vi "Create_Raw_data_file.vi"(4 "No of averages":i32=1, 5 "End time":dbl, 6 "Start time":dbl, 7 "Setup filename":string) -> (0 "Error String":string, 1 "Values":string[][](array[string]), 2 "Header Comments":string[](array[string]), 3 "Column headers":string[](array[string]))   [LabVIEW 2011]
uses:
  File/Setup_Filetype.ctl
  Controls/Post_Process.ctl
  Globals/Preference_global.vi
  Globals/Meas_global.vi
  Globals/Trav_pos_global.vi
  Globals/Constants_global.vi
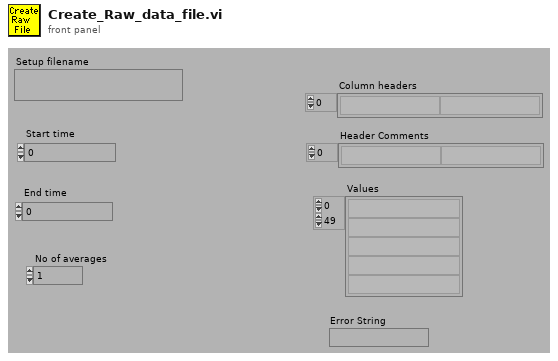
[diagram p1: front panel]
types:
  T1 = typedef "Post_Process.ctl" = enum16{"Take New Data", "Post Process Raw Data File"}
  T2 = typedef "Server_Comms.ctl" = enum16{"Server Link Healthy", "Do Not Link To Server"}
  T3 = typedef "Setup_Filetype.ctl" = enum16{"Measurement Setups", "Calibration Setups", "General", "Results File Plotter Setups", "Speed Calib Tweaks"}
  T4 = typedef "Traverse_cluster.ctl" = cluster{"Start X":dbl, "Start Y":dbl, "Start Z":dbl, "End X":dbl, "End Y":dbl, "End Z":dbl, "No. of pts.":i32, "Spacing":T5, "Filename":path, "Tunnel Speed":dbl, "Averaging time (min)":dbl, "Extra Commands":string, "Specific Arguments":string, "Emission Rate (l/min)":dbl, "Trace Gas Concentration (%)":dbl, "Density Ratio":string, "Comments":string, "Row No":i32, "Row Type Selector":T6, "Completion time":string, "Row Duration (mins)":dbl, "No. of Valid pts.":i32, "Meas Setup File":string}
  T5 = typedef "Spacing.ctl" = enum16{"Linear", "Log", "Gauss", "Specified", "N/A"}
  T6 = typedef "Multi_run_mode.ctl" = enum16{"Move Traverse Only", "Set Tunnel Speed Only", "Set Source Only", "Set Measurement Conditions", "Single Measurement", "Vertical Profile", "Lateral Profile", "Longitudinal Profile", "Explore Volume", "Multi-Axis Profile", "Auto Calibrate", "Meas Fast FID Bkgnd", "Check Beam Power", "Scanning Valve Measurement", "Run VI Named:", "Set ADAM Ch", "Wait (minutes)", "Send Message", "Synchronize With:", "Fall Back to this Row", "Turn Off Row Repeating", "Blank Row", "Traverse 3D Volume"}
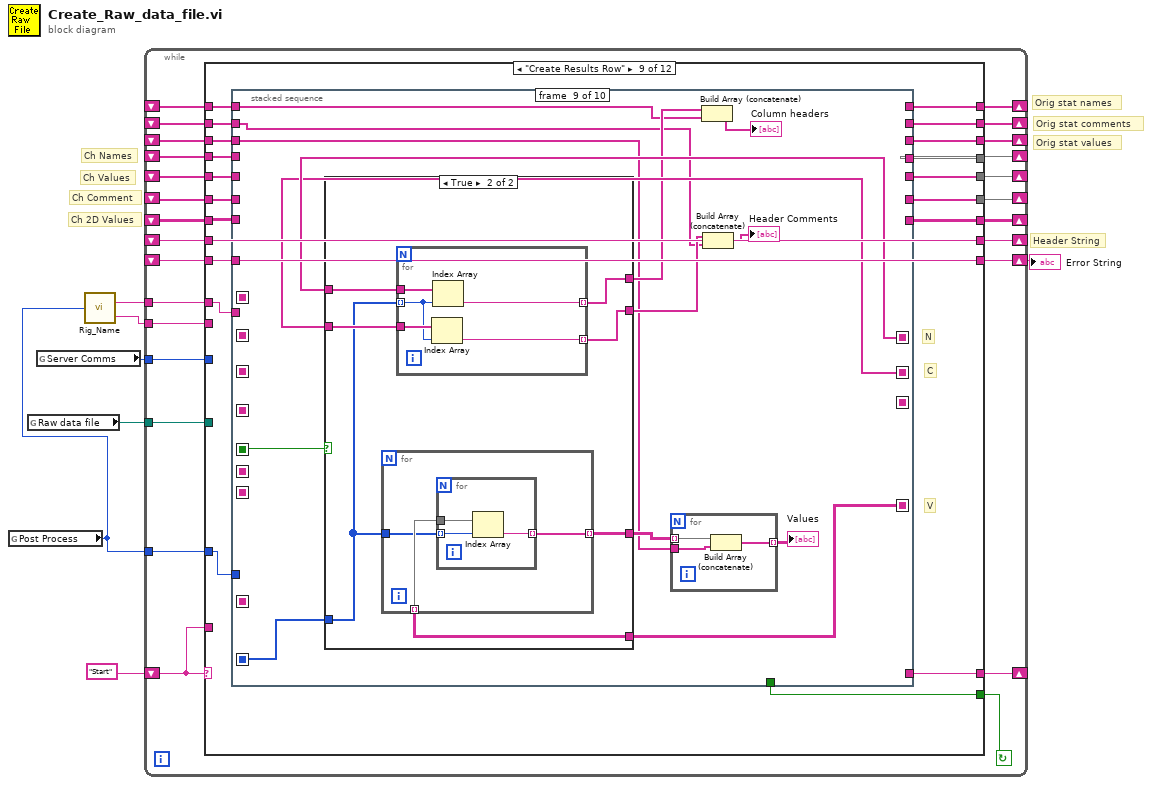
[diagram p0: block diagram]
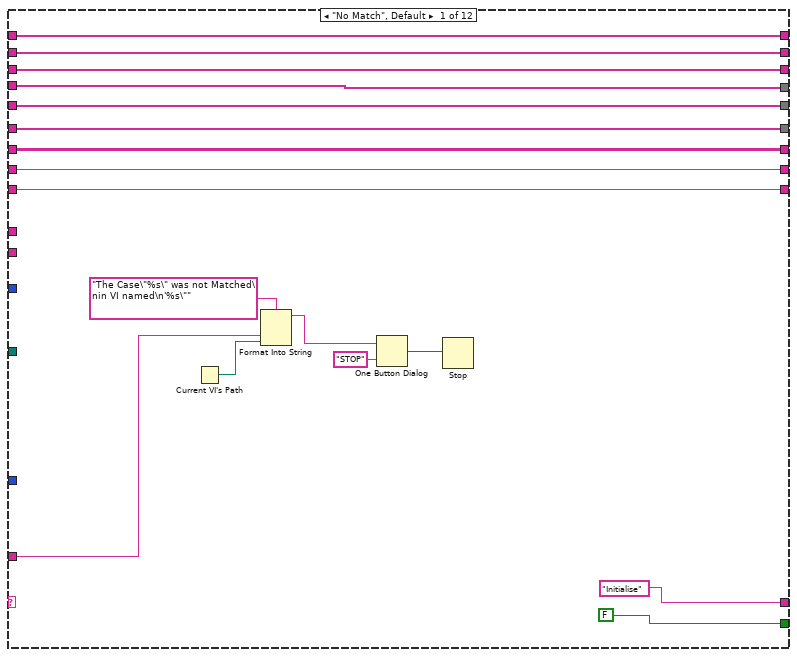
[diagram p2: hidden frame]
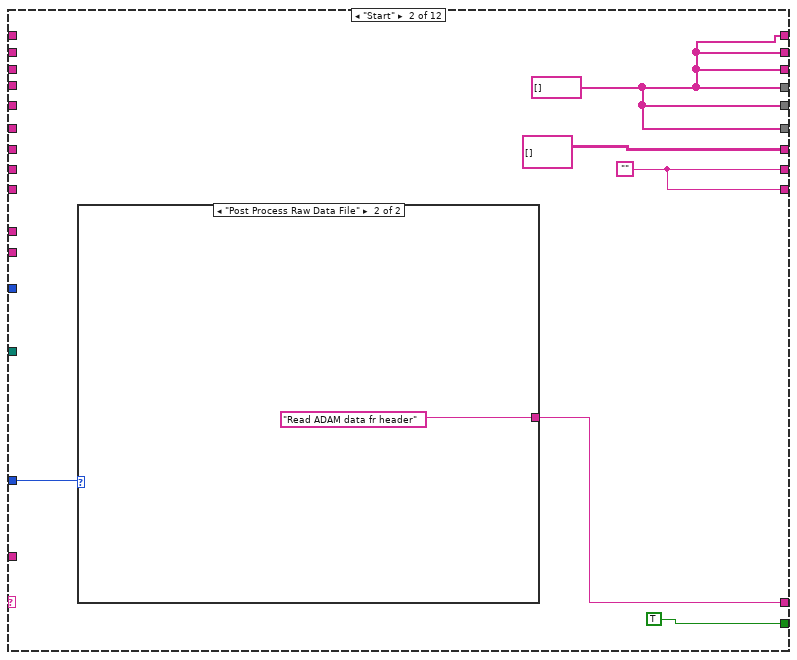
[diagram p3: hidden frame]
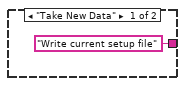
[diagram p4: hidden frame]
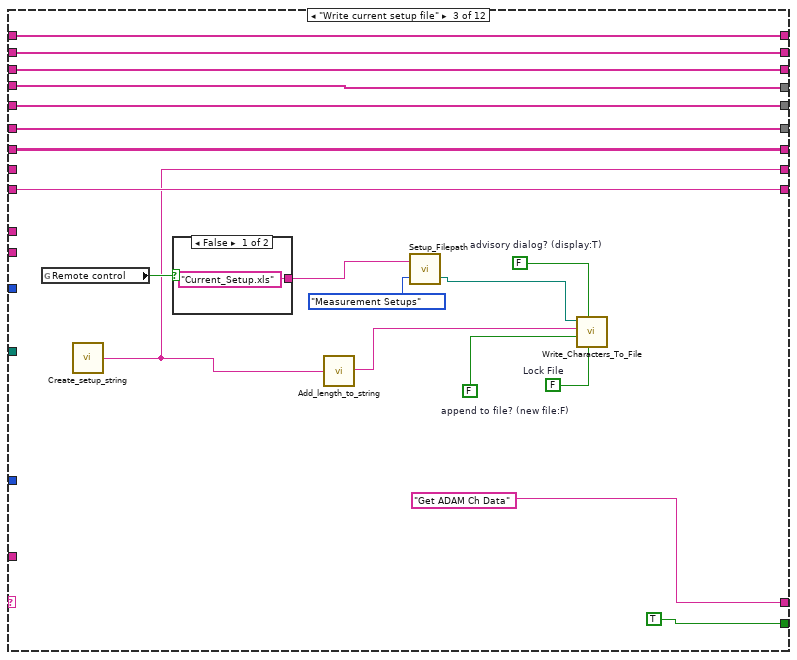
[diagram p5: hidden frame]
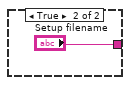
[diagram p6: hidden frame]
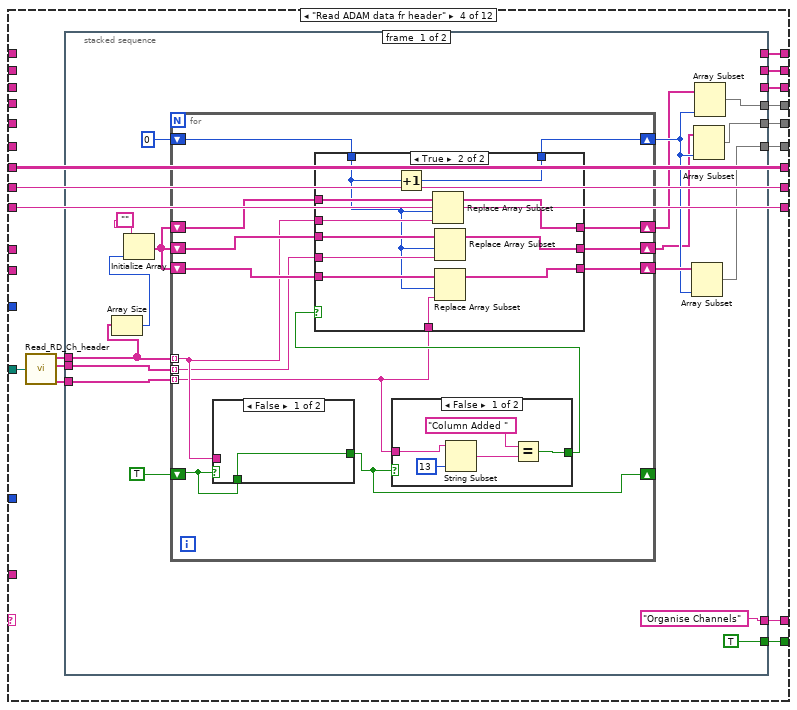
[diagram p7: hidden frame]
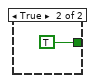
[diagram p9: hidden frame]
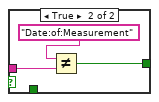
[diagram p10: hidden frame]
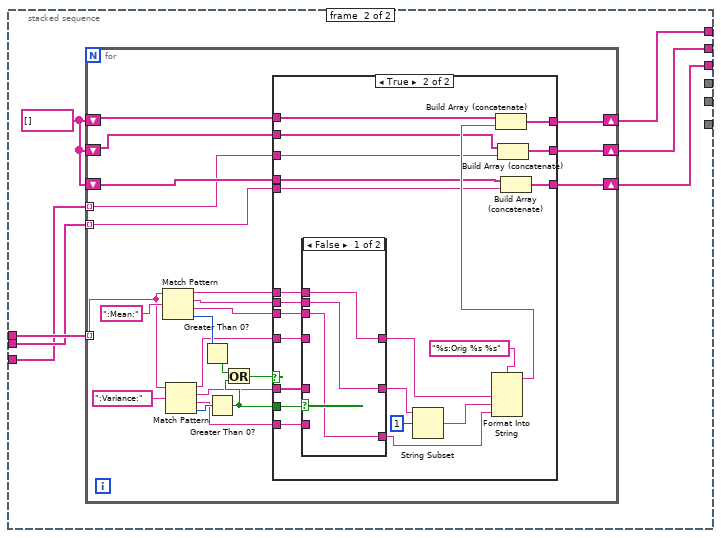
[diagram p11: hidden frame]
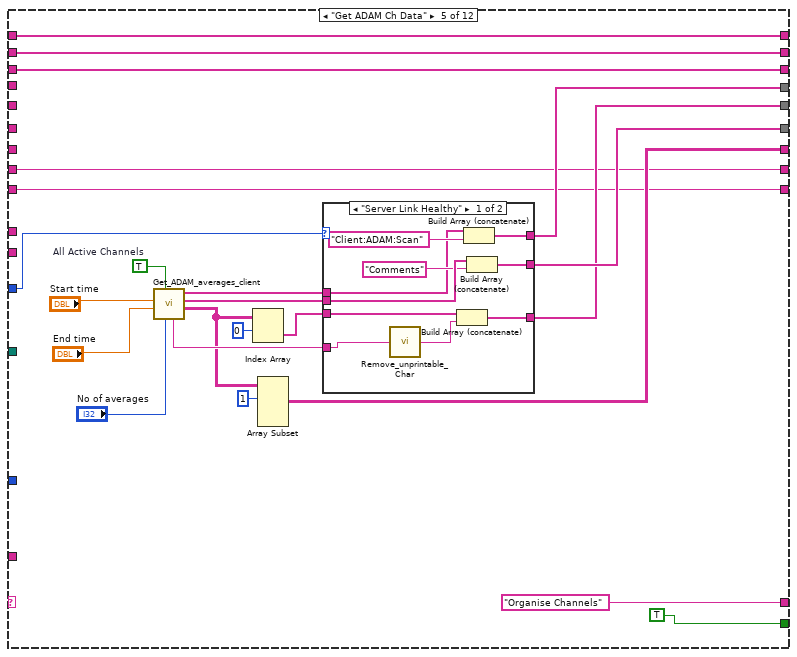
[diagram p14: hidden frame]
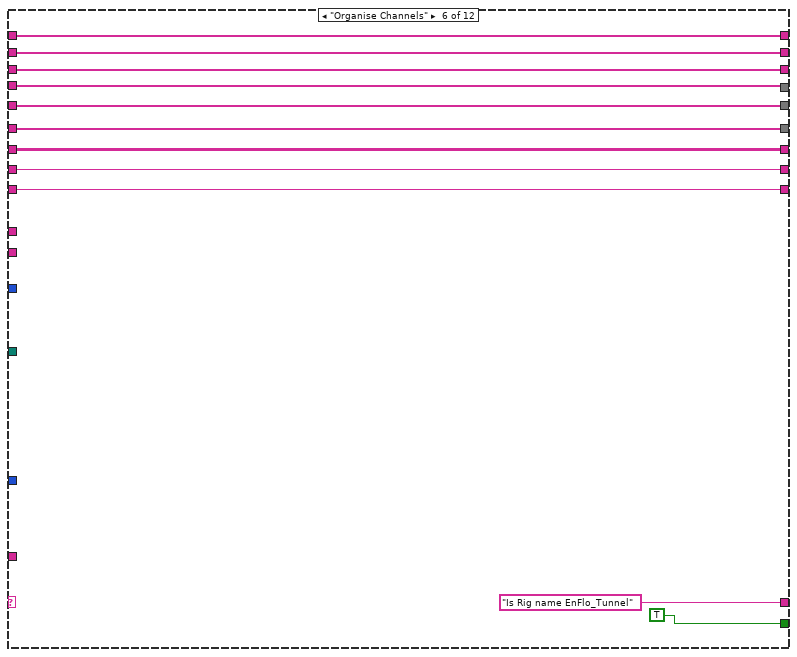
[diagram p16: hidden frame]
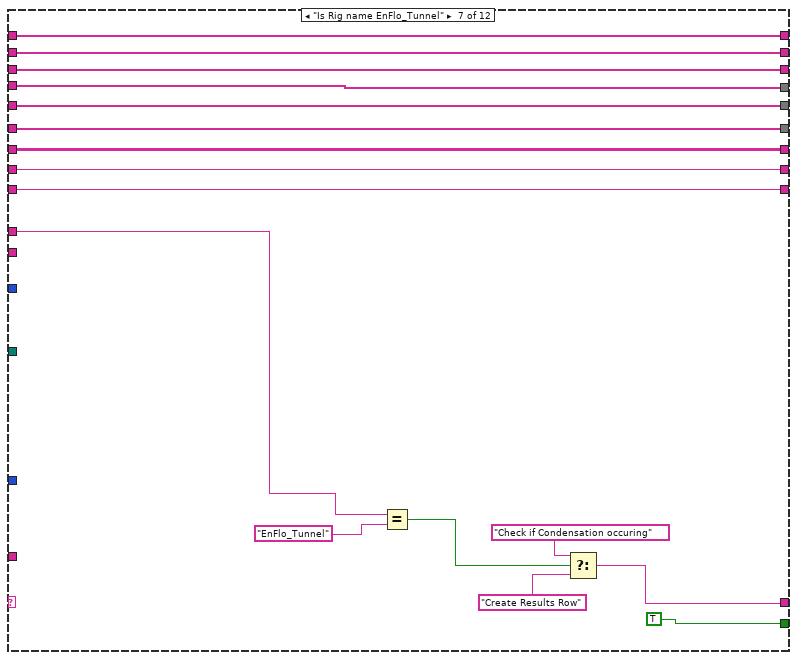
[diagram p17: hidden frame]
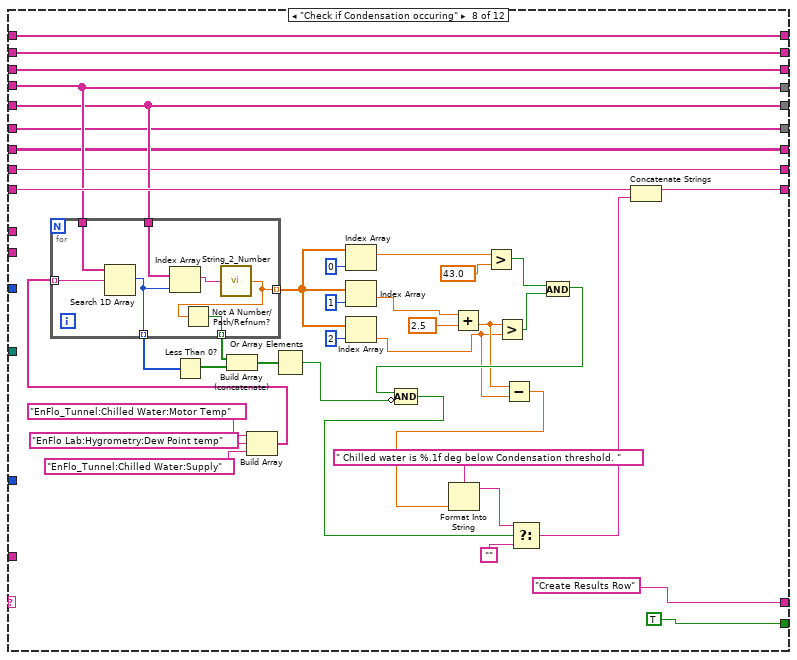
[diagram p18: hidden frame]
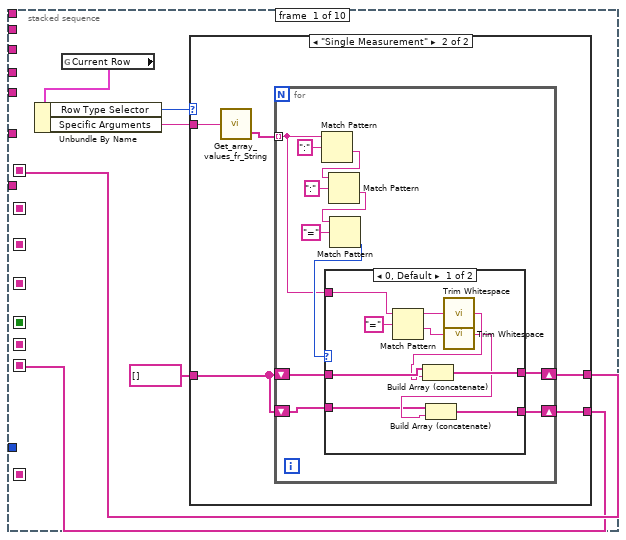
[diagram p19: hidden frame]
diagram:
  # "Orig stat values"
  # "Orig stat comments"
  # "Orig stat names"
  # "Header String"
  # "Ch 2D Values"
  # "Ch Comment"
  # "Ch Values"
  # "Ch Names"
  n1 = global read "Meas_global.vi" "Post Process"() -> (w3:T1)
  n2 = global read "Meas_global.vi" "Raw data file"() -> (w6:path)
  n3 = global read "Preference_global.vi" "Server Comms"() -> (w5:T2)
  n4 = call "Rig_Name.vi"("Post Process"=w3) -> ("Rig Setup before dash"=w2:string, "Hard Disk name"=w1:string)
  n5 = while {
    tunnel: w5 -> [w16]
    tunnel: w6 -> [w17]
    tunnel: w3 -> [w18]
    shift-left: _ -> [w20]
    shift-right: [w19] -> _
    shift-left: _ -> [w26]
    shift-right: [w25] -> w4
    shift-left: _ -> [w21]
    shift-right: [w27] -> _
    shift-left: _ -> [w22]
    shift-right: [w29] -> _
    shift-left: _ -> [w23]
    shift-right: [w28] -> _
    shift-left: _ -> [w24]
    shift-right: [w30] -> _
    shift-left: "Start" -> [w31]
    shift-right: [w32] -> _
    tunnel: w2 -> [w15]
    tunnel: w1 -> [w14]
    shift-right: [w10] -> _
    shift-left: _ -> [w11]
    shift-right: [w8] -> _
    shift-left: _ -> [w9]
    shift-right: [w12] -> _
    shift-left: _ -> [w13]
    stop <- w33 continue-if-true
    n6 = case shown="\"Create Results Row\"" w31 {
      tunnel: [FALSE TRUE TRUE w83 TRUE TRUE TRUE TRUE w328 TRUE TRUE FALSE] -> w33
      tunnel: ["Initialise" w52 "Get ADAM Ch Data" w94 "Organise Channels" "Is Rig name EnFlo_Tunnel" w265 "Create Results Row" w340 "Add Raw Data header info" "Add Raw Data fr Tempory file" "End"] -> w32
      tunnel: w31 -> [w45 _ _ _ _ _ _ _ _ _ _ _]
      tunnel: [w42 w51 w77 w85 w221 w255 w273 w283 w337 w625 w655 w672] -> w30
      tunnel: [w40 w51 w75 w86 w220 w253 w271 w281 w334 w636 w657 w674] -> w29
      tunnel: [w41 w51 w76 w84 w219 w254 w272 w282 w330 w637 w656 w673] -> w28
      tunnel: [w39 string[][] [] w74 w92 w217 w252 w270 w280 w332 w628 w658 w675] -> w27
      tunnel: w26 -> [w38 _ w72 w93 w216 w250 w267 w286 w338 w641 w659 w676]
      tunnel: [w38 w54 w72 w93 w216 w250 w267 w284 w338 w641 w659 w676] -> w25
      tunnel: w24 -> [w42 _ w77 _ _ w255 w273 w283 w336 w625 w655 w672]
      tunnel: w23 -> [w41 _ w76 _ _ w254 w272 w282 w331 w637 w656 w673]
      tunnel: w22 -> [w40 _ w75 _ _ w253 w271 w281 w335 w636 w657 w674]
      tunnel: w21 -> [w39 _ w74 w92 _ w252 w270 w280 w333 w628 w658 w675]
      tunnel: w20 -> [w37 _ _ w91 w215 w251 w268 w278 w339 w630 w652 w671]
      tunnel: [w37 w54 w66 w91 w215 w251 w268 w278 w339 w633 w651 ""] -> w19
      tunnel: w18 -> [_ w53 _ _ _ _ _ _ w329 _ _ _]
      tunnel: w17 -> [_ _ _ w90 _ _ _ _ _ _ _ w667]
      tunnel: w16 -> [_ _ _ _ w214 _ _ _ _ _ _ _]
      tunnel: w15 -> [_ _ _ _ _ _ w262 _ w327 _ _ _]
      tunnel: w14 -> [_ _ _ _ _ _ _ _ _ _ _ _]
      tunnel: w13 -> [w36 _ w64 _ w213 w249 w260 w277 w325 w622 w650 w664]
      tunnel: [w36 w51 w64 w82 w213 w249 w260 w277 w326 w622 w650 w664] -> w12
      tunnel: w11 -> [w35 _ w63 _ w212 w248 w259 w276 w324 w621 w649 w663]
      tunnel: [w35 w51 w63 w81 w212 w248 w259 w276 w323 w621 w649 w663] -> w10
      tunnel: w9 -> [w34 _ w62 _ w211 w247 w258 w275 w321 w620 w648 w662]
      tunnel: [w34 w51 w62 w80 w211 w247 w258 w275 w322 w620 w648 w662] -> w8
      frame "No Match", Default {
        n7 = Current VI's Path() -> (path=w44:path)
        n8 = Format Into String(format string="The Case\"%s\" was not Matched\nin VI named\n'%s\"" ("Format String"), w45, w44) -> (resulting string=w48:string)  [unwired: 2 in, 1 out]
        n9 = One Button Dialog(message=w48, button name ("OK")="STOP") -> (true=w46:bool)
        n10 = Stop(stop? (T)=w46) -> ()
      }
      frame "Start" {
        w54 = ""
        w51 = string[] []
        n11 = case shown="\"Post Process Raw Data File\"" w53 {
          tunnel: ["Write current setup file" "Read ADAM data fr header"] -> w52
          frame "Take New Data" {
          }
          frame "Post Process Raw Data File" {
          }
        }
      }
      frame "Write current setup file" {
        w67 = FALSE  # Lock File
        w70 = FALSE  # advisory dialog? (display:T)
        w71 = FALSE  # append to file? (new file:F)
        n12 = global read "Meas_global.vi" "Remote control"() -> (w69:bool)
        n13 = call "Create_setup_string.vi"() -> ("Setup String"=w66:string)  [unwired: 1 out]
        n14 = case shown="False" w69 {
          tunnel: ["Current_Setup.xls" ("Setup filename") "Setup filename"] -> w60
          frame False {
          }
          frame True {
          }
        }
        n15 = call "Add_length_to_string.vi"("String in"=w66) -> ("String out"=w68:string)
        n16 = call "Setup_Filepath.vi"("Setup File Type"=Setup_Filetype."Measurement Setups", "Filename in"=w60) -> ("Filename Out"=w59:path)  [unwired: 1 out]
        n17 = call "Write_Characters_To_File.vi"("file path (dialog if empty)"=w59, "advisory dialog? (display:T)"=w70, "character string"=w68, "append to file? (new file:F)"=w71, "Lock File"=w67) -> ()  [unwired: 4 out]
      }
      frame "Read ADAM data fr header" {
        n18 = call "Read_RD_Ch_header.vi"("Raw data file"=w90) -> ("Ch Name Out"=w88:string[], "Ch Values"=w87:string[], "Comments"=w89:string[])  [unwired: 1 out]
        n19 = stacked-sequence {
          tunnel: ["Organise Channels" _] -> w94
          tunnel: w89 -> [w109 w154]
          tunnel: w88 -> [w108 w157]
          tunnel: w87 -> [w103 w155]
          tunnel: [w100 _] -> w86
          tunnel: [w97 _] -> w85
          tunnel: [w96 _] -> w84
          tunnel: [TRUE _] -> w83
          tunnel: [_ w153] -> w82
          tunnel: [_ w152] -> w81
          tunnel: [_ w151] -> w80
          frame #0 {
            n20 = Array Size(array=w108) -> (size(s)=w106:i32)
            n21 = Initialize Array("", w106) -> (w105:string[])
            n22 = for {
              shift-right: [w112] -> w101
              shift-left: 0 -> [w122]
              shift-right: [w116] -> w102
              shift-left: w105 -> [w119]
              shift-right: [w117] -> w99
              shift-left: w105 -> [w120]
              shift-right: [w118] -> w98
              shift-left: w105 -> [w121]
              shift-right: [w124] -> _
              shift-left: TRUE -> [w125]
              tunnel: w108 -> [w115] mode=indexing
              tunnel: w109 -> [w113] mode=indexing
              tunnel: w103 -> [w114] mode=indexing
              n23 = case shown="False" w125 {
                tunnel: w115 -> [_ w150]
                tunnel: [w147 w148] -> w124
                tunnel: w125 -> [w147 _]
                frame False {
                }
                frame True {
                  n24 = Not Equal?(x="Date:of:Measurement", y=w150) -> (x != y?=w148:bool)
                }
              }
              n25 = case shown="False" w124 {
                tunnel: w113 -> [w142 _]
                tunnel: [w144 TRUE] -> w123
                frame False {
                  n26 = String Subset(string=w142, length (rest)=13 ("length (rest)")) -> (substring=w141:string)  [unwired: 1 out]
                  n27 = Equal?(x="Column Added ", y=w141) -> (x = y?=w144:bool)
                }
                frame True {
                }
              }
              n28 = case shown="True" w123 {
                tunnel: w122 -> [w126 w131]
                tunnel: w121 -> [w129 w140]
                tunnel: w120 -> [w128 w139]
                tunnel: w119 -> [w127 w138]
                tunnel: [w129 w137] -> w118
                tunnel: [w128 w136] -> w117
                tunnel: [w127 w135] -> w116
                tunnel: w115 -> [_ w134]
                tunnel: w114 -> [_ w133]
                tunnel: w113 -> [_ w132]
                tunnel: [w126 w130] -> w112
                frame False {
                }
                frame True {
                  n29 = Increment(x=w131) -> (x+1=w130:i32)
                  n30 = Replace Array Subset(array=w140, new element=w134, index=w131) -> (w137:string[])
                  n31 = Replace Array Subset(array=w139, new element=w133, index=w131) -> (w136:string[])
                  n32 = Replace Array Subset(array=w138, new element=w132, index=w131) -> (w135:string[])
                }
              }
            }
            n33 = Array Subset(array=w102, length=w101) -> (w100:string[])  [unwired: 1 in]
            n34 = Array Subset(array=w99, length=w101) -> (w96:string[])  [unwired: 1 in]
            n35 = Array Subset(array=w98, length=w101) -> (w97:string[])  [unwired: 1 in]
          }
          frame #1 {
            w156 = string[] []
            n36 = for {
              shift-right: [w165] -> w153
              shift-left: w156 -> [w164]
              shift-right: [w158] -> w152
              shift-left: w156 -> [w159]
              shift-right: [w161] -> w151
              shift-left: w156 -> [w162]
              tunnel: w157 -> [w177] mode=indexing
              tunnel: w155 -> [w163] mode=indexing
              tunnel: w154 -> [w160] mode=indexing
              n37 = Match Pattern(string=w177, regular expression=":Mean:") -> (before substring=w168:string, match substring=w167:string, after substring=w166:string, offset past match=w176:i32)  [unwired: 1 out]
              n38 = Match Pattern(string=w177, regular expression=":Variance:") -> (before substring=w171:string, match substring=w170:string, after substring=w169:string, offset past match=w175:i32)  [unwired: 1 out]
              n39 = Greater Than 0?(x=w176) -> (x > 0?=w174:bool)
              n40 = Greater Than 0?(x=w175) -> (x > 0?=w172:bool)
              n41 = Or(x=w174, y=w172) -> (x .or. y?=w173:bool)
              n42 = case shown="True" w173 {
                tunnel: w172 -> [_ w204]
                tunnel: w171 -> [_ w203]
                tunnel: w170 -> [_ w202]
                tunnel: w169 -> [_ w201]
                tunnel: w168 -> [_ w194]
                tunnel: w167 -> [_ w193]
                tunnel: w166 -> [_ w192]
                tunnel: [w182 w190] -> w165
                tunnel: w164 -> [w182 w189]
                tunnel: w163 -> [_ w188]
                tunnel: w162 -> [w180 w187]
                tunnel: [w180 w186] -> w161
                tunnel: w160 -> [_ w185]
                tunnel: w159 -> [w181 w184]
                tunnel: [w181 w183] -> w158
                frame False {
                }
                frame True {
                  n43 = case shown="False" w204 {
                    tunnel: w203 -> [_ w209]
                    tunnel: w202 -> [_ w210]
                    tunnel: w201 -> [_ w208]
                    tunnel: [w206 w210] -> w199
                    tunnel: [w207 w209] -> w196
                    tunnel: [w205 w208] -> w195
                    tunnel: w194 -> [w207 _]
                    tunnel: w193 -> [w206 _]
                    tunnel: w192 -> [w205 _]
                    frame False {
                    }
                    frame True {
                    }
                  }
                  n44 = String Subset(string=w199, offset (0)=1) -> (substring=w198:string)  [unwired: 1 out]
                  n45 = Format Into String(format string="%s:Orig %s %s", w196, w198, w195) -> (resulting string=w191:string)  [unwired: 2 in, 1 out]
                  n46 = Build Array (concatenate)(w189, w191) -> (w190:string[])
                  n47 = Build Array (concatenate)(w184, w185) -> (w183:string[])
                  n48 = Build Array (concatenate)(w187, w188) -> (w186:string[])
                }
              }
            }
          }
        }
      }
      frame "Get ADAM Ch Data" {
        w224 = TRUE  # All Active Channels
        n49 = call "Get_ADAM_averages_client.vi"("No of averages"="No of averages", "All Active Channels"=w224, "End time"="End time", "Start time"="Start time") -> ("Values"=w227:string[][], "Comments"=w230:string[], "Titles"=w229:string[], "Messages"=w231:string)  [unwired: 1 in, 3 out]
        n50 = Index Array(array=w227, index (row)=0 ("Index")) -> (element=w218:string[])  [unwired: 1 in]
        n51 = Array Subset(array=w227, index (row)=1 ("Array Index")) -> (w217:string[][])  [unwired: 3 in]
        n52 = case shown="\"Server Link Healthy\"" w214 {
          tunnel: w231 -> [w235 _]
          tunnel: w230 -> [w243 w245]
          tunnel: w229 -> [w240 w246]
          tunnel: [w239 w246] -> w221
          tunnel: [w238 w245] -> w220
          tunnel: [w237 w244] -> w219
          tunnel: w218 -> [w236 w244]
          frame "Server Link Healthy" {
            n53 = call "Remove_unprintable_Char.vi"("Input String"=w235) -> ("Output String"=w234:string)
            n54 = Build Array (concatenate)(w236, w234) -> (w237:string[])
            n55 = Build Array (concatenate)(w240, "Client:ADAM:Scan") -> (w239:string[])
            n56 = Build Array (concatenate)(w243, "Comments" ("Comments")) -> (w238:string[])
          }
          frame "Do Not Link To Server" {
          }
        }
      }
      frame "Organise Channels" {
      }
      frame "Is Rig name EnFlo_Tunnel" {
        n57 = Equal?(x=w262, y="EnFlo_Tunnel") -> (x = y?=w266:bool)
        n58 = Select(t="Check if Condensation occuring", s=w266, f="Create Results Row") -> (s? t:f=w265:string)
      }
      frame "Check if Condensation occuring" {
        n59 = Build Array("EnFlo_Tunnel:Chilled Water:Motor Temp", "EnFlo Lab:Hygrometry:Dew Point temp", "EnFlo_Tunnel:Chilled Water:Supply") -> (w309:string[])
        n60 = for {
          tunnel: w283 -> [w320]
          tunnel: w309 -> [w319] mode=indexing
          tunnel: w282 -> [w318]
          tunnel: [w316] -> w310 mode=indexing
          tunnel: [w315] -> w308 mode=indexing
          tunnel: [w314] -> w301 mode=indexing
          n61 = Search 1D Array(1D array=w320, element=w319) -> (index of element=w316:i32)  [unwired: 1 out]
          n62 = Index Array(array=w318, index=w316) -> (element=w317:string)
          n63 = call "String_2_Number.vi"("Value"=w317) -> ("Numeric"=w315:dbl)
          n64 = Not A Number/Path/Refnum?(number/path/refnum=w315) -> (NaN/Path/Refnum?=w314:bool)
        }
        n65 = Less Than 0?(x=w310) -> (x < 0?=w300:bool[])
        n66 = Build Array (concatenate)(w301, w300) -> (w299:bool[])
        n67 = Or Array Elements(Boolean array=w299) -> (logical OR=w295:bool)
        n68 = Index Array(array=w308, index=0 ("Index")) -> (element=w302:dbl)
        n69 = Index Array(array=w308, index=1 ("Index")) -> (element=w298:dbl)
        n70 = Index Array(array=w308, index=2 ("Index")) -> (element=w290:dbl)
        n71 = Add(x=w298, y=2.5) -> (x+y=w291:dbl)
        n72 = Greater?(x=w302, y=43.0) -> (0:w296:bool)
        n73 = Greater?(x=w291, y=w290) -> (0:w297:bool)
        n74 = Subtract(x=w291, y=w290) -> (x-y=w289:dbl)
        n75 = Format Into String(format string=" Chilled water is %.1f deg below Condensation threshold. " ("Format String"), w289) -> (resulting string=w287:string)  [unwired: 2 in, 1 out]
        n76 = And(x=w296, y=w297) -> (x .and. y?=w294:bool)
        n77 = Compound Arithmetic op=AND(w294, invert w295) -> (w293:bool)
        n78 = Select(t=w287, s=w293, f="") -> (s? t:f=w285:string)
        n79 = Concatenate Strings(w286, w285) -> (w284:string)
      }
      frame "Create Results Row" {
        # "V"
        # "C"
        # "N"
        n80 = stacked-sequence {
          seq-local: [_ w378 _ _ _ _ _ _ _ _] -> [_ _ _ w420 w461 _ _ _ _ _]
          seq-local: [_ w377 _ _ _ _ _ _ _ _] -> [_ _ _ w416 w460 _ _ _ _ _]
          seq-local: [_ _ w400 _ _ _ _ _ _ _] -> [_ _ _ w414 w459 _ _ _ _ _]
          seq-local: [_ w385 _ _ _ _ _ _ _ _] -> [_ _ _ _ _ w496 _ _ _ _]
          seq-local: [_ _ _ _ w458 _ _ _ _ _] -> [_ _ _ _ _ w498 _ _ _ _]
          seq-local: [w342 _ _ _ _ _ _ _ _ _] -> [_ w381 _ _ _ _ _ _ _ _]
          seq-local: [w341 _ _ _ _ _ _ _ _ _] -> [_ _ w402 _ _ _ _ _ _ _]
          seq-local: [_ _ _ _ w457 _ _ _ _ _] -> [_ _ _ _ _ _ _ w553 w591 _]
          seq-local: [_ _ _ _ w456 _ _ _ _ _] -> [_ _ _ _ _ _ _ _ w589 _]
          seq-local: [_ _ _ _ _ w495 _ _ _ _] -> [_ _ _ _ _ _ _ _ w588 _]
          seq-local: [_ _ _ _ _ _ w513 _ _ _] -> [_ _ _ _ _ _ _ w552 w592 _]
          seq-local: [_ _ _ _ _ _ _ w551 _ _] -> [_ _ _ _ _ _ _ _ w590 _]
          seq-local: [_ w376 _ _ _ _ _ _ _ _] -> [_ _ w401 _ _ _ _ _ _ _]
          tunnel: [_ _ "Add Adam Chs to header" _ _ _ _ _ _ _] -> w340
          tunnel: w336 -> [_ w384 _ w418 _ _ w516 _ _ _]
          tunnel: w335 -> [_ w383 _ w419 _ _ _ _ _ _]
          tunnel: w338 -> [_ _ w405 _ _ _ _ _ _ _]
          tunnel: w331 -> [_ _ w404 w413 _ _ w515 _ _ _]
          tunnel: w333 -> [_ _ w403 _ _ _ _ _ _ _]
          tunnel: [_ _ _ w417 _ _ _ _ _ _] -> w337
          tunnel: [_ _ _ w415 _ _ _ _ _ _] -> w334
          tunnel: [_ _ w403 _ _ _ _ _ _ _] -> w332
          tunnel: [_ _ _ w412 _ _ _ _ _ _] -> w330
          tunnel: w329 -> [_ _ _ w411 w462 _ w523 _ _ _]
          tunnel: [_ _ _ _ _ _ w519 _ _ _] -> w328
          tunnel: w327 -> [_ _ _ _ _ _ w517 _ _ _]
          tunnel: [_ _ _ _ _ _ _ _ _ w619] -> w326
          tunnel: w325 -> [_ _ _ _ _ _ _ _ w586 w619]
          tunnel: w324 -> [_ _ _ _ _ _ _ _ w583 w618]
          tunnel: [_ _ _ _ _ _ _ _ _ w618] -> w323
          tunnel: [_ _ _ _ _ _ _ _ _ w617] -> w322
          tunnel: w321 -> [_ _ _ _ _ _ _ _ w580 w617]
          frame #0 {
            n81 = global read "Trav_pos_global.vi" "Current Row"() -> (w346:T4)
            n82 = Unbundle By Name(w346) -> ("Row Type Selector"=w345:T6, "Specific Arguments"=w344:string)
            n83 = case shown="\"Single Measurement\"" w345 {
              tunnel: w344 -> [_ w352]
              tunnel: string[] [] -> [w347 w350]
              tunnel: [w347 w349] -> w342
              tunnel: [w347 w348] -> w341
              frame "Move Traverse Only", Default {
              }
              frame "Single Measurement" {
                n84 = call "Get_array_values_fr_String.vi"("String Value"=w352) -> ("String array"=w351:string[])  [unwired: 1 out]
                n85 = for {
                  tunnel: w351 -> [w355] mode=indexing
                  shift-right: [w353] -> w348
                  shift-left: w350 -> [w354]
                  shift-right: [w356] -> w349
                  shift-left: w350 -> [w357]
                  n86 = Match Pattern(string=w355, regular expression=":") -> (after substring=w361:string)  [unwired: 4 out]
                  n87 = Match Pattern(string=w361, regular expression=":") -> (after substring=w359:string)  [unwired: 4 out]
                  n88 = Match Pattern(string=w359, regular expression="=") -> (offset past match=w358:i32)  [unwired: 4 out]
                  n89 = case shown="0, Default" w358 {
                    tunnel: w357 -> [w373 w375]
                    tunnel: [w372 w375] -> w356
                    tunnel: w355 -> [w368 _]
                    tunnel: w354 -> [w365 w374]
                    tunnel: [w364 w374] -> w353
                    frame 0, Default {
                      n90 = Match Pattern(string=w368, regular expression="=") -> (before substring=w370:string, after substring=w369:string)  [unwired: 3 out]
                      n91 = call <vilib>:"Trim Whitespace.vi"("string"=w370) -> ("trimmed string"=w367:string)  [unwired: 1 in]
                      n92 = Build Array (concatenate)(w373, w367) -> (w372:string[])
                      n93 = call <vilib>:"Trim Whitespace.vi"("string"=w369) -> ("trimmed string"=w366:string)  [unwired: 1 in]
                      n94 = Build Array (concatenate)(w365, w366) -> (w364:string[])
                    }
                    frame -1 {
                    }
                  }
                }
              }
            }
          }
          frame #1 {
            n95 = for {
              tunnel: w384 -> [w398] mode=indexing
              tunnel: w383 -> [w397] mode=indexing
              tunnel: [w396] -> w380 mode=indexing
              n96 = Concatenate Strings(w398, ":" ("Substring"), w397) -> (w396:string)
            }
            n97 = call "Create_Results_Row.vi"() -> ("row splitting"=w385:string[][], "Channel Values"=w376:string[], "Channel Names"=w382:string[])  [unwired: 3 in]
            n98 = Build Array (concatenate)(w382, w381, w380) -> (w379:string[])
            n99 = for {
              tunnel: w379 -> [w386] mode=indexing
              tunnel: [w390] -> w378 mode=indexing
              tunnel: [w387] -> w377 mode=indexing
              w389 = ":" ("regular expression")
              n100 = Match Pattern(string=w386, regular expression=w389) -> (before substring=w393:string, after substring=w395:string)  [unwired: 3 out]
              n101 = Match Pattern(string=w395, regular expression=w389) -> (before substring=w392:string, after substring=w394:string)  [unwired: 3 out]
              n102 = Match Pattern(string=w394, regular expression=w389) -> (before substring=w391:string, after substring=w388:string)  [unwired: 3 out]
              n103 = Match Pattern(string=w388, regular expression=w389) -> (before substring=w387:string)  [unwired: 4 out]
              n104 = Concatenate Strings(w393, w389, w392, w389, w391) -> (w390:string)
            }
          }
          frame #2 {
            w406 = 5  # Comment Column
            n105 = Index Array(array=w401, index=w406) -> (element=w408:string)
            n106 = Concatenate Strings(w408, w405) -> (w409:string)
            n107 = Replace Array Subset(array=w401, new element=w409, index=w406) -> (w407:string[])
            n108 = Build Array (concatenate)(w407, w402, w404) -> (w400:string[])
          }
          frame #3 {
            n109 = case shown="\"Take New Data\"" w411 {
              tunnel: w420 -> [w429 _]
              tunnel: w419 -> [w428 w454]
              tunnel: w418 -> [w427 w455]
              tunnel: [w426 w455] -> w417
              tunnel: w416 -> [w425 _]
              tunnel: [w424 w454] -> w415
              tunnel: w414 -> [w423 _]
              tunnel: w413 -> [w422 w453]
              tunnel: [w421 w453] -> w412
              frame "Take New Data" {
                n110 = for {
                  tunnel: w427 -> [w440]
                  tunnel: w429 -> [w436] mode=indexing
                  shift-right: [w437] -> w426
                  shift-left: w427 -> [w438]
                  shift-right: [w434] -> w424
                  shift-left: w428 -> [w435]
                  shift-right: [w431] -> w421
                  shift-left: w422 -> [w432]
                  tunnel: w425 -> [w433] mode=indexing
                  tunnel: w423 -> [w430] mode=indexing
                  n111 = Search 1D Array(1D array=w440, element=w436) -> (index of element=w439:i32)  [unwired: 1 out]
                  n112 = case shown="-1" w439 {
                    tunnel: w438 -> [w443 w452]
                    tunnel: [w443 w450] -> w437
                    tunnel: w436 -> [_ w451]
                    tunnel: w435 -> [w442 w449]
                    tunnel: [w442 w448] -> w434
                    tunnel: w433 -> [_ w447]
                    tunnel: w432 -> [w441 w445]
                    tunnel: [w441 w444] -> w431
                    tunnel: w430 -> [_ w446]
                    frame 0, Default {
                    }
                    frame -1 {
                      n113 = Build Array (concatenate)(w445, w446) -> (w444:string[])
                      n114 = Build Array (concatenate)(w452, w451) -> (w450:string[])
                      n115 = Build Array (concatenate)(w449, w447) -> (w448:string[])
                    }
                  }
                }
              }
              frame "Post Process Raw Data File" {
              }
            }
          }
          frame #4 {
            # "Values"
            # "Comments"
            # "Ch Names"
            n116 = case shown="\"Post Process Raw Data File\"" w462 {
              tunnel: [w465 w471] -> w457
              tunnel: w461 -> [w465 w472]
              tunnel: [w464 w470] -> w456
              tunnel: w460 -> [w464 w468]
              tunnel: [w463 w469] -> w458
              tunnel: w459 -> [w463 w467]
              frame "Take New Data" {
              }
              frame "Post Process Raw Data File" {
                w466 = string[] []
                n117 = for {
                  shift-right: [w480] -> w471
                  shift-left: w466 -> [w481]
                  shift-right: [w475] -> w470
                  shift-left: w466 -> [w478]
                  shift-right: [w476] -> w469
                  shift-left: w466 -> [w477]
                  tunnel: w472 -> [w479] mode=indexing
                  tunnel: w468 -> [w474] mode=indexing
                  tunnel: w467 -> [w473] mode=indexing
                  n118 = Search 1D Array(1D array=w481, element=w479) -> (index of element=w482:i32)  [unwired: 1 out]
                  n119 = case shown="-1" w482 {
                    tunnel: w481 -> [w485 w494]
                    tunnel: [w485 w493] -> w480
                    tunnel: w479 -> [_ w492]
                    tunnel: w478 -> [w484 w491]
                    tunnel: w477 -> [w483 w490]
                    tunnel: [w483 w489] -> w476
                    tunnel: [w484 w488] -> w475
                    tunnel: w474 -> [_ w487]
                    tunnel: w473 -> [_ w486]
                    frame 0, Default {
                    }
                    frame -1 {
                      n120 = Build Array (concatenate)(w494, w492) -> (w493:string[])
                      n121 = Build Array (concatenate)(w491, w487) -> (w488:string[])
                      n122 = Build Array (concatenate)(w490, w486) -> (w489:string[])
                    }
                  }
                }
              }
            }
          }
          frame #5 {
            n123 = Array Size(array=w496) -> (size(s)=w501:i32[])
            n124 = Index Array(array=w501, index=0) -> (element=w499:i32)
            n125 = Greater Than 0?(x=w499) -> (x > 0?=w497:bool)
            n126 = case shown="True" w497 {
              tunnel: w498 -> [w503 w507]
              tunnel: w496 -> [_ w505]
              tunnel: [w502 w504] -> w495
              frame False {
                n127 = Build Array(w503) -> (w502:string[][])
              }
              frame True {
                n128 = Search 1D Array(1D array=w507, element="Instrument_name_place_holder") -> (index of element=w506:i32)  [unwired: 1 out]
                n129 = for {
                  tunnel: w507 -> [w512]
                  tunnel: w506 -> [w511]
                  tunnel: w505 -> [w510] mode=indexing
                  tunnel: [w509] -> w504 mode=indexing
                  n130 = Replace Array Subset(array=w512, new element=w510, index=w511) -> (w509:string[])
                }
              }
            }
          }
          frame #6 {
            n131 = Equal?(x="EnFlo_Tunnel", y=w517) -> (x = y?=w514:bool)
            n132 = case shown="True" w514 {
              tunnel: w516 -> [_ w532]
              tunnel: w515 -> [_ w529]
              tunnel: [FALSE w527] -> w513
              frame False {
              }
              frame True {
                n133 = disable-structure shown="Enabled" {
                  disable-tunnel: [w533 FALSE] -> w525
                  frame Disabled {
                    n134 = global read "Meas_global.vi" "Pre Setup String"() -> (w537:string)
                    n135 = call "Get_Characters_from_string.vi"("Input string"=w537, "Variable name"="Show_all_EnFlo_Tunnel_Columns") -> ("Status"=w535:enum16{"Char in string", "Char not in string"}, "Value"=w534:string)  [unwired: 1 in]
                    n136 = case shown="\"Char in string\"" w535 {
                      tunnel: w534 -> [w540 _]
                      tunnel: [w538 TRUE] -> w533
                      frame "Char in string" {
                        n137 = Equal?(x=w540, y="TRUE") -> (x = y?=w539:bool)
                        n138 = Not(x=w539) -> (.not. x?=w538:bool)
                      }
                      frame "Char not in string" {
                      }
                    }
                  }
                  frame Enabled {
                  }
                }
                n139 = Search 1D Array(1D array=w532, element="EnFlo_Tunnel:Heater:Enable") -> (index of element=w530:i32)  [unwired: 1 out]
                n140 = case shown="-1" w530 {
                  tunnel: w530 -> [w549 _]
                  tunnel: w529 -> [w548 _]
                  tunnel: [w544 FALSE] -> w528
                  frame 0, Default {
                    n141 = Index Array(array=w548, index=w549) -> (element=w547:string)
                    n142 = call "String_2_Number.vi"("Value"=w547) -> ("Numeric"=w546:dbl)
                    n143 = Less?(x=w546, y=0.5) -> (x < y?=w544:bool)
                  }
                  frame -1 {
                  }
                }
                n144 = Select(t=w528, s=w525, f=FALSE) -> (s? t:f=w527:bool)
              }
            }
            n145 = global read "Trav_pos_global.vi" "Dummy Measurement?"() -> (w520:bool)
            n146 = Equal?(x=Post_Process."Take New Data" ("Post Process"), y=w523) -> (x = y?=w521:bool)
            n147 = Compound Arithmetic op=AND(invert w520, w521) -> (w519:bool)
          }
          frame #7 {
            n148 = case shown="True" w552 {
              tunnel: w553 -> [_ w559]
              tunnel: [i32[] [] w557] -> w551
              frame False {
              }
              frame True {
                w555 = string[] ["EnFlo_Tunnel:Inlet Heater:Temp", "EnFlo_Tunnel:Inlet Rake:Temp", "EnFlo_Tunnel:Trav Thermo:", "EnFlo_Tunnel:floor ", "EnFlo_Tunnel:roof ", "EnFlo_Tunnel:Side ", "EnFlo_Tunnel:Temp:Inlet", "EnFlo_Tunnel:Temp:Floor"] ("Column headers")
                # "Remove these\nChannels"
                # "Remaining\nChannels"
                n149 = for {
                  tunnel: w555 -> [w561] mode=indexing
                  tunnel: [w560] -> w556 mode=indexing
                  n150 = String Length(string=w561) -> (length=w560:i32)
                }
                n151 = for {
                  tunnel: w559 -> [w565] mode=indexing
                  shift-right: [w568] -> w557
                  shift-left: i32[] [] -> [w569]
                  tunnel: w556 -> [w566]
                  tunnel: w555 -> [w564]
                  i -> [w567]
                  n152 = for {
                    tunnel: w566 -> [w574] mode=indexing
                    tunnel: w565 -> [w573]
                    tunnel: w564 -> [w571] mode=indexing
                    tunnel: [w570] -> w563 mode=indexing
                    n153 = String Subset(string=w573, length (rest)=w574) -> (substring=w572:string)  [unwired: 1 out]
                    n154 = Equal?(x=w572, y=w571) -> (x = y?=w570:bool)
                  }
                  n155 = Or Array Elements(Boolean array=w563) -> (logical OR=w562:bool)
                  n156 = case shown="True" w562 {
                    tunnel: w569 -> [w577 w578]
                    tunnel: w567 -> [w576 _]
                    tunnel: [w575 w578] -> w568
                    frame False {
                      n157 = Build Array (concatenate)(w577, w576) -> (w575:i32[])
                    }
                    frame True {
                    }
                  }
                }
              }
            }
          }
          frame #8 {
            n158 = case shown="True" w592 {
              tunnel: w591 -> [w598 w605]
              tunnel: w590 -> [_ w600]
              tunnel: w589 -> [w597 w604]
              tunnel: [w598 w603] -> w587
              tunnel: [w597 w602] -> w584
              tunnel: w588 -> [w596 w601]
              tunnel: [w596 w599] -> w581
              frame False {
              }
              frame True {
                n159 = for {
                  tunnel: w601 -> [w608] mode=indexing
                  tunnel: w600 -> [w607]
                  tunnel: [w606] -> w599 mode=indexing
                  n160 = for {
                    tunnel: w608 -> [w610]
                    tunnel: w607 -> [w611] mode=indexing
                    tunnel: [w609] -> w606 mode=indexing
                    n161 = Index Array(array=w610, index=w611) -> (element=w609:string)
                  }
                }
                n162 = for {
                  tunnel: w605 -> [w616]
                  tunnel: w600 -> [w612] mode=indexing
                  tunnel: w604 -> [w615]
                  tunnel: [w614] -> w603 mode=indexing
                  tunnel: [w613] -> w602 mode=indexing
                  n163 = Index Array(array=w615, index=w612) -> (element=w613:string)
                  n164 = Index Array(array=w616, index=w612) -> (element=w614:string)
                }
              }
            }
            n165 = for {
              tunnel: w581 -> [w595] mode=indexing
              tunnel: w580 -> [w594]
              tunnel: [w593] -> w579 mode=indexing
              n166 = Build Array (concatenate)(w595, w594) -> (w593:string[])
            }
            "Values" <- w579
            n167 = Build Array (concatenate)(w587, w586) -> (→"Column headers":string[])
            n168 = Build Array (concatenate)(w584, w583) -> (→"Header Comments":string[])
          }
          frame #9 {
          }
        }
      }
      frame "Add Adam Chs to header" {
        w623 = FALSE  # Email On Error?
        n169 = call "Channel_name_checker.vi"("Email On Error?"=w623, "Channel names"=w625) -> ("Channel names Out"=w624:string[])  [unwired: 1 out]
        n170 = for {
          tunnel: w624 -> [w647] mode=indexing
          tunnel: [w646] -> w640 mode=indexing
          tunnel: [w645] -> w639 mode=indexing
          tunnel: [w644] -> w638 mode=indexing
          n171 = call "Split_Ch_name.vi"("Ch name"=w647) -> ("Top level"=w646:string, "Middle"=w645:string, "Low level"=w644:string)
        }
        n172 = Array To Spreadsheet String(array=w628, 3:"%s" ("format string")) -> (spreadsheet string=w626:string)  [unwired: 1 out]
        n173 = Build Array(w640, w639, w638, w637, w636) -> (w634:string[][])
        n174 = Array To Spreadsheet String(array=w634, 3:"%s" ("format string")) -> (spreadsheet string=w627:string)  [unwired: 1 out]
        n175 = Concatenate Strings(w627, w626, "***************************************" ("Substring"), "\r", w630) -> (w633:string)
      }
      frame "Add Raw Data header info" {
        n176 = String Length(string=w652) -> (length=w654:i32)
        n177 = call "Raw_Data_File_Start_text.vi"("Header length"=w654) -> ("Start String"=w653:string)
        n178 = Concatenate Strings(w653, w652) -> (w651:string)
      }
      frame "Add Raw Data fr Tempory file" {
        w665 = 0  # Start to copy file at:
        n179 = global read "Constants_global.vi" "Data Folder Local"() -> (w669:path)
        n180 = Build Path(base path=w669, name or relative path="Tempory_Raw_Data_File.xls") -> (appended path=w666:path)
        n181 = call "Piece_file_Copy.vi"("File Start String"=w671, "Start to copy file at:"=w665, "Source File"=w666, "Target File"=w667) -> ()  [unwired: 1 out]
      }
    }
  }
  "Error String" <- w4
